vi "StopTarget.vi"(11 "DCM Reference":refnum<class "DCM - RT.lvclass">) -> (3 "Stop":bool)   [LabVIEW 2015, in "DSI-RT.lvlib"]
uses:
  <vilib>/Powertrain Controls/Device Drivers/DCM/Rev0/RT/DCM - RT.lvclass
  <vilib>/Powertrain Controls/Device Drivers/DCM/Rev0/RT/DCM - RT.lvclass/DCM - RT.ctl
  <vilib>/Powertrain Controls/Device Drivers/DCM/Rev0/RT/Read Stop Target.vi
  DSI-RT.lvlib
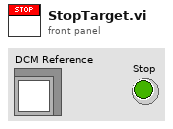
[diagram p1: front panel]
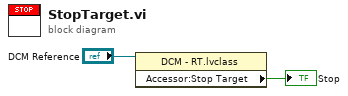
[diagram p0: block diagram]
diagram:
  n1 = property class="DCM - RT.lvclass"(reference="DCM Reference") -> ("Accessor:Stop Target"=→"Stop":bool)  [unwired: 1 in, 2 out]
